vi "_Load All Tables.vi"(7 "Use temporary file (F)":bool) -> (2 "ADC Table":T1[](array[typedef]), 3 "Loaded ADC":bool)   [LabVIEW 2015]
uses:
  Type/_RT Configuration 2.ctl
  Type/_RT Command.ctl
  Configuration/_Global Configuration.vi
  <vilib>/Utility/config.llb/Write Key (String).vi
  <vilib>/Utility/config.llb/NI_LVConfig.lvlib
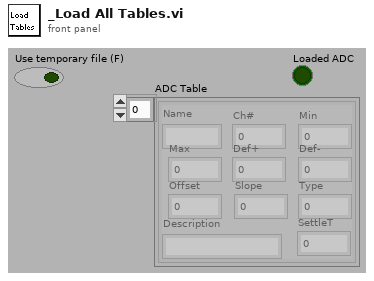
[diagram p1: front panel]
types:
  T1 = typedef "_RT Configuration 2.ctl" = cluster{"Name":string, "Ch#":u8, "Min":dbl, "Max":dbl, "Def+":dbl, "Def-":dbl, "Offset":dbl, "Slope":dbl, "Type":u8, "Description":string, "SettleT":dbl}
  T2 = enum32{"existing file", "new file", "new or existing file", "existing dir", "new dir", "new or existing dir", "existing file (use LLBs)", "new file (use LLBs)", "new or existing file (use LLBs)", "new or existing file or directory (use LLBs)"}
  T3 = typedef "_RT Command.ctl" = enum16{"Start", "Stop", "Runtime Update", "Get Data", "Get Info", "Get Status", "Get Param", "Get Config", "Get Table", "Read ADC", "Set Oscillator", "Update Config", "Update Table", "Set All Pol", "Set Pol and DC", "Set Max Mass", "Toggle RP", "Toggle EL", "Set PIC", "Initialize Turbo", "Send Turbo Comm", "Close Turbo", "P1", "P2", "P3", "Send Serial", "Set LC Out", "Get LC In", "Read VAC", "Test Table", "Toggle Power", "Get Startup", "Set Startup", "Get ADC Table", "Set ADC Table", "Get Brief Status", "Get Detail Status", "Auxiliary Update", "Set CC Logics", "Set CC Input Logics", "Ignore Error"}
  T4 = typedef "_RT Instrument 2.ctl" = cluster{"Table":T1[], "Instrument":string[]}
  T5 = typedef "NI_LVConfig.lvlib/Config Data RefNum.ctl" = refnum<k1>
  T6 = typedef "_Instrument Model.ctl" = enum16{"IONICS 3QA", "IONICS 3QB", "IONICS 3Q 110", "IONICS 3Q 120", "IONICS 3Q 210", "IONICS 3Q 220", "IONICS 3Q 310", "IONICS 3Q 320", "SHIMADZU LCMS-8080", "Simulation (Single Source)", "Simulation (Dual Source)"}
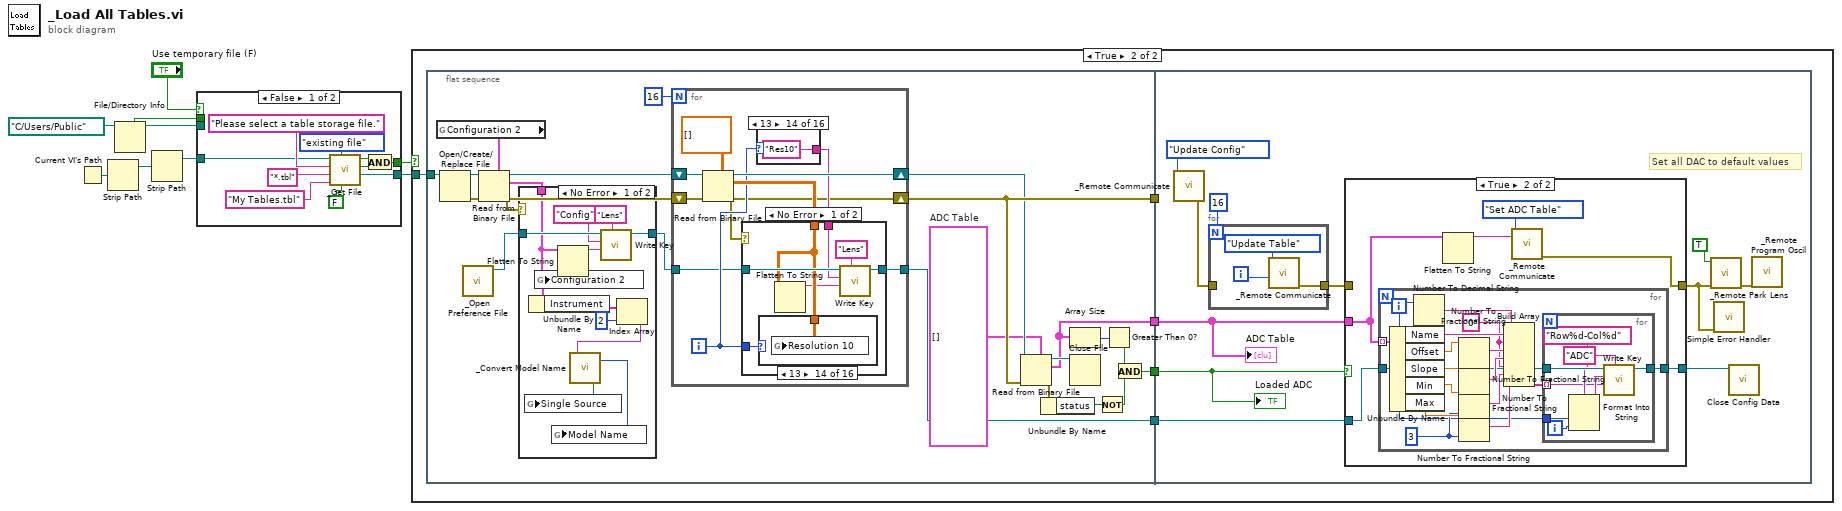
[diagram p0: block diagram]
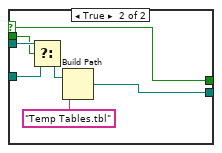
[diagram p2: hidden frame]
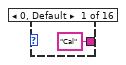
[diagram p4: hidden frame]
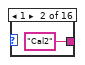
[diagram p5: hidden frame]
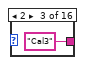
[diagram p6: hidden frame]
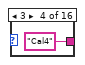
[diagram p7: hidden frame]
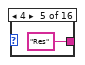
[diagram p8: hidden frame]
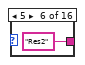
[diagram p9: hidden frame]
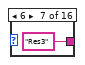
[diagram p10: hidden frame]
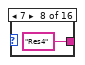
[diagram p11: hidden frame]
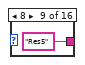
[diagram p12: hidden frame]
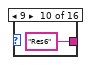
[diagram p13: hidden frame]
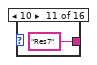
[diagram p14: hidden frame]
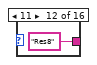
[diagram p15: hidden frame]
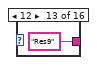
[diagram p16: hidden frame]
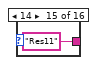
[diagram p17: hidden frame]
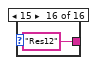
[diagram p18: hidden frame]
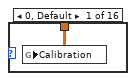
[diagram p19: hidden frame]
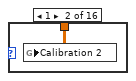
[diagram p20: hidden frame]
diagram:
  n1 = Current VI's Path() -> (path=w8:path)
  n2 = Strip Path(path=w8) -> (stripped path=w9:path)  [unwired: 1 out]
  n3 = File/Directory Info(path=path "C:/Users/Public" ("stripped path")) -> (path out=w1:path, directory=w2:bool)  [unwired: 1 in, 5 out]
  n4 = Strip Path(path=w9) -> (stripped path=w7:path)  [unwired: 1 out]
  n5 = case shown="False" "Use temporary file (F)" {
    selector: "Use temporary file (F)" -> [_ w24]
    tunnel: w7 -> [w13 w22]
    tunnel: [w12 w25] -> w6
    tunnel: [w11 w24] -> w5
    tunnel: w2 -> [_ w21]
    tunnel: w1 -> [_ w23]
    frame False {
      n6 = call "_Get File.vi"("For Write (T)"=FALSE, "select mode (new or existing)"=T2."existing file", "default name"="My Tables.tbl", "extension (isd)"="*.tbl" ("pattern (all files)"), "prompt"="Please select a table storage file.", "Start Path"=w13) -> ("Seleted File"=w12:path, "Exists"=w19:bool, "Succeeded"=w18:bool)  [unwired: 1 out]
      n7 = And(x=w18, y=w19) -> (x .and. y?=w11:bool)
    }
    frame True {
      n8 = Select(t=w23, s=w21, f=w22) -> (s? t:f=w20:path)
      n9 = Build Path(base path=w20, name or relative path="Temp Tables.tbl") -> (appended path=w25:path)
    }
  }
  n10 = case shown="True" w5 {
    tunnel: w6 -> [_ w31]
    frame False {
    }
    frame True {
      n11 = flat-sequence {
        tunnel: w31 -> [w50]
        tunnel: [w43] -> w30
        tunnel: [w34] -> w29
        tunnel: [w33] -> w28
        tunnel: [w32] -> w27
        tunnel: w30 -> [_]
        tunnel: w29 -> [w121]
        tunnel: w28 -> [w118]
        tunnel: w27 -> [w117]
        frame #0 {
          w40 = T1[] []  # ADC Table
          n12 = global read "_Global Configuration.vi" "Configuration 2"() -> (w49:T4)
          n13 = Open/Create/Replace File(file path (use dialog)=w50) -> (refnum out=w51:refnum<file>, error out=w52:errorcluster)  [unwired: 5 in, 1 out]
          n14 = call "_Open Preference File.vi"() -> ("refnum"=w53:T5)  [unwired: 1 in, 6 out]
          n15 = Read from Binary File(5:w49, 8:w52, 11:w51) -> (0:w45:errorcluster, 2:w48:T4, 3:w46:refnum<file>)  [unwired: 4 out]
          n16 = case shown="No Error" w45 {
            tunnel: w53 -> [w114 w115]
            tunnel: w48 -> [w107 _]
            tunnel: [w110 w115] -> w47
            frame No Error {
              n17 = Unbundle By Name(w107) -> ("Instrument"=w109:string[])
              n18 = global write "_Global Configuration.vi" "Configuration 2"(w107) -> ()
              n19 = Flatten To String(anything=w107) -> (data string=w111:string)  [unwired: 1 in, 4 out]
              n20 = call-poly <vilib>:"Write Key.vi"("section"="Lens", "value"=w111, "key"="Config" ("section"), "refnum"=w114) -> ("refnum out"=w110:T5)  [unwired: 2 in, 5 out]
              n21 = Index Array(array=w109, index=2) -> (element=w106:string)
              n22 = call "_Convert Model Name.vi"("Model"=w106) -> ("SingleSource"=w105:bool, "Model Name"=w104:T6)  [unwired: 1 in]
              n23 = global write "_Global Configuration.vi" "Single Source"(w105) -> ()
              n24 = global write "_Global Configuration.vi" "Model Name"(w104) -> ()
            }
            frame Error {
            }
          }
          n25 = for {
            N: 16 -> [_]
            tunnel: w47 -> [w57]
            shift-right: [w59] -> w42
            shift-left: w46 -> [w63]
            shift-right: [w55] -> w43
            shift-left: w45 -> [w62]
            tunnel: [w54] -> w32
            i -> [w58]
            n26 = Read from Binary File(5:dbl[][] [] ("Cal-"), 8:w62, 11:w63) -> (0:w55:errorcluster, 2:w60:dbl[][], 3:w59:refnum<file>)  [unwired: 4 out]
            n27 = case shown="13" w58 {
              tunnel: ["Cal" ("section") "Cal2" ("section") "Cal3" ("section") "Cal4" ("section") "Res" ("section") "Res2" ("section") "Res3" ("section") "Res4" ("section") "Res5" ("section") "Res6" ("section") "Res7" ("section") "Res8" ("section") "Res9" ("section") "Res10" ("section") "Res11" ("section") "Res12" ("section")] -> w56
              frame 0, Default {
              }
              frame 1 {
              }
              frame 2 {
              }
              frame 3 {
              }
              frame 4 {
              }
              frame 5 {
              }
              frame 6 {
              }
              frame 7 {
              }
              frame 8 {
              }
              frame 9 {
              }
              frame 10 {
              }
              frame 11 {
              }
              frame 12 {
              }
              frame 13 {
              }
              frame 14 {
              }
              frame 15 {
              }
            }
            n28 = case shown="No Error" w55 {
              tunnel: w60 -> [w82 _]
              tunnel: w58 -> [w86 _]
              tunnel: w57 -> [w85 w103]
              tunnel: w56 -> [w83 _]
              tunnel: [w80 w103] -> w54
              frame No Error {
                n29 = case shown="13" w86 {
                  tunnel: w82 -> [w87 w88 w89 w90 w91 w92 w93 w94 w95 w96 w97 w98 w99 w100 w101 w102]
                  frame 0, Default {
                    n30 = global write "_Global Configuration.vi" "Calibration"(w87) -> ()
                  }
                  frame 1 {
                    n31 = global write "_Global Configuration.vi" "Calibration 2"(w88) -> ()
                  }
                  frame 2 {
                    n32 = global write "_Global Configuration.vi" "Calibration 3"(w89) -> ()
                  }
                  frame 3 {
                    n33 = global write "_Global Configuration.vi" "Calibration 4"(w90) -> ()
                  }
                  frame 4 {
                    n34 = global write "_Global Configuration.vi" "Resolution"(w91) -> ()
                  }
                  frame 5 {
                    n35 = global write "_Global Configuration.vi" "Resolution 2"(w92) -> ()
                  }
                  frame 6 {
                    n36 = global write "_Global Configuration.vi" "Resolution 3"(w93) -> ()
                  }
                  frame 7 {
                    n37 = global write "_Global Configuration.vi" "Resolution 4"(w94) -> ()
                  }
                  frame 8 {
                    n38 = global write "_Global Configuration.vi" "Resolution 5"(w95) -> ()
                  }
                  frame 9 {
                    n39 = global write "_Global Configuration.vi" "Resolution 6"(w96) -> ()
                  }
                  frame 10 {
                    n40 = global write "_Global Configuration.vi" "Resolution 7"(w97) -> ()
                  }
                  frame 11 {
                    n41 = global write "_Global Configuration.vi" "Resolution 8"(w98) -> ()
                  }
                  frame 12 {
                    n42 = global write "_Global Configuration.vi" "Resolution 9"(w99) -> ()
                  }
                  frame 13 {
                    n43 = global write "_Global Configuration.vi" "Resolution 10"(w100) -> ()
                  }
                  frame 14 {
                    n44 = global write "_Global Configuration.vi" "Resolution 11"(w101) -> ()
                  }
                  frame 15 {
                    n45 = global write "_Global Configuration.vi" "Resolution 12"(w102) -> ()
                  }
                }
                n46 = Flatten To String(anything=w82) -> (data string=w81:string)  [unwired: 1 in, 4 out]
                n47 = call-poly <vilib>:"Write Key.vi"("section"="Lens", "value"=w81, "key"=w83, "refnum"=w85) -> ("refnum out"=w80:T5)  [unwired: 2 in, 5 out]
              }
              frame Error {
              }
            }
          }
          n48 = Read from Binary File(5:w40, 8:w43, 11:w42) -> (0:w38:errorcluster, 2:w33:T1[], 3:w41:refnum<file>)  [unwired: 4 out]
          n49 = Unbundle By Name(w38) -> ("status"=w37:bool)
          n50 = Array Size(array=w33) -> (size(s)=w39:i32)
          n51 = Close File(refnum=w41) -> ()  [unwired: 1 in, 2 out]
          n52 = Not(x=w37) -> (.not. x?=w35:bool)
          n53 = Greater Than 0?(x=w39) -> (x > 0?=w36:bool)
          n54 = And(x=w36, y=w35) -> (x .and. y?=w34:bool)
        }
        frame #1 {
          # "Set all DAC to default values"
          n55 = call "_Remote Communicate.vi"("Command"=_RT_Command."Update Config") -> ("error out"=w122:errorcluster)  [unwired: 5 in, 3 out]
          n56 = for {
            N: 16 -> [_]
            tunnel: w122 -> [_]
            tunnel: [w161] -> w120
            i -> [w160]
            n57 = call "_Remote Communicate.vi"("DC Param"=w160, "Command"=_RT_Command."Update Table") -> ("error out"=w161:errorcluster)  [unwired: 4 in, 3 out]
          }
          n58 = case shown="True" w121 {
            tunnel: w120 -> [w128 _]
            tunnel: [w128 w133] -> w119
            tunnel: w118 -> [_ w131]
            tunnel: w117 -> [w127 w130]
            tunnel: [w127 w129] -> w116
            frame False {
            }
            frame True {
              n59 = for {
                tunnel: w131 -> [w151] mode=indexing
                tunnel: w130 -> [w138]
                tunnel: [w135] -> w129
                i -> [w137]
                w141 = "0"
                w146 = i16 3 ("precision (6)")
                n60 = Unbundle By Name(w151) -> ("Name"=w144:string, "Offset"=w150:dbl, "Slope"=w149:dbl, "Min"=w148:dbl, "Max"=w147:dbl)
                n61 = Number To Decimal String(number=w137) -> (decimal integer string=w145:string)  [unwired: 1 out]
                n62 = Number To Fractional String(number=w150) -> (F-format string=w143:string)  [unwired: 3 out]
                n63 = Number To Fractional String(number=w149) -> (F-format string=w142:string)  [unwired: 3 out]
                n64 = Number To Fractional String(number=w148, precision (6)=w146) -> (F-format string=w140:string)  [unwired: 2 out]
                n65 = Number To Fractional String(number=w147, precision (6)=w146) -> (F-format string=w139:string)  [unwired: 2 out]
                n66 = Build Array(w145, w144, w141, w143, w142, w141, w140, w139) -> (w136:string[])
                n67 = for {
                  tunnel: w138 -> [w159]
                  tunnel: w137 -> [w157]
                  tunnel: w136 -> [w153] mode=indexing
                  tunnel: [w152] -> w135
                  i -> [w158]
                  n68 = Format Into String(format string="Row%d-Col%d" ("section"), w157, w158) -> (resulting string=w155:string)  [unwired: 2 in, 1 out]
                  n69 = call-poly <vilib>:"Write Key.vi"("section"="ADC", "value"=w153, "key"=w155, "refnum"=w159) -> ("refnum out"=w152:T5)  [unwired: 2 in, 5 out]
                }
              }
              n70 = Flatten To String(anything=w131) -> (data string=w132:string)  [unwired: 1 in, 4 out]
              n71 = call "_Remote Communicate.vi"("String"=w132, "Command"=_RT_Command."Set ADC Table") -> ("error out"=w133:errorcluster)  [unwired: 4 in, 3 out]
            }
          }
          n72 = call "_Remote Park Lens.vi"("error in"=w119, "All Ch (F)"=TRUE) -> ("error out"=w123:errorcluster)  [unwired: 5 out]
          n73 = call <vilib>:"Simple Error Handler.vi"("error in (no error)"=w119) -> ()  [unwired: 1 in, 8 out]
          n74 = call <vilib>:"Close Config Data.vi"("refnum"=w116) -> ()  [unwired: 2 in, 9 out]
          n75 = call "_Remote Program Oscil.vi"("error in (no error)"=w123) -> ()  [unwired: 1 out]
          "Loaded ADC" <- w121
          "ADC Table" <- w118
        }
      }
    }
  }
